vi "PID Test.vi"() -> ()   [LabVIEW 2017]
uses:
  <vilib>/addons/control/pid/NI_PID_pid.lvlib
  <vilib>/addons/control/pid/pid.llb/PID (DBL).vi
  <vilib>/myRIO/Instrument Drivers/Utilities/Utilities.lvlib
panel:
  out "Time (s)":dbl
  out "Output String":string
  out "PID Output":dbl(graph)
  out "SP & PV":T1(graph)
  out "Speed (mm/s)":dbl
  in  "PID gains":T2={"proportional gain (Kc)"=1.0, "integral time (Ti, min)"=0.01, "derivative time (Td, min)"=0.0} {"derivative time (Td, min)" format="%.3f"; "integral time (Ti, min)" format="%.3f"; "proportional gain (Kc)" format="%.3f"}
  out "dt out (s)":dbl format="%.3f"
  in  "FWD/RVS":bool
  in  "Frequency":dbl
  in  "Velocity Set Pt":dbl
  in  "stop":bool
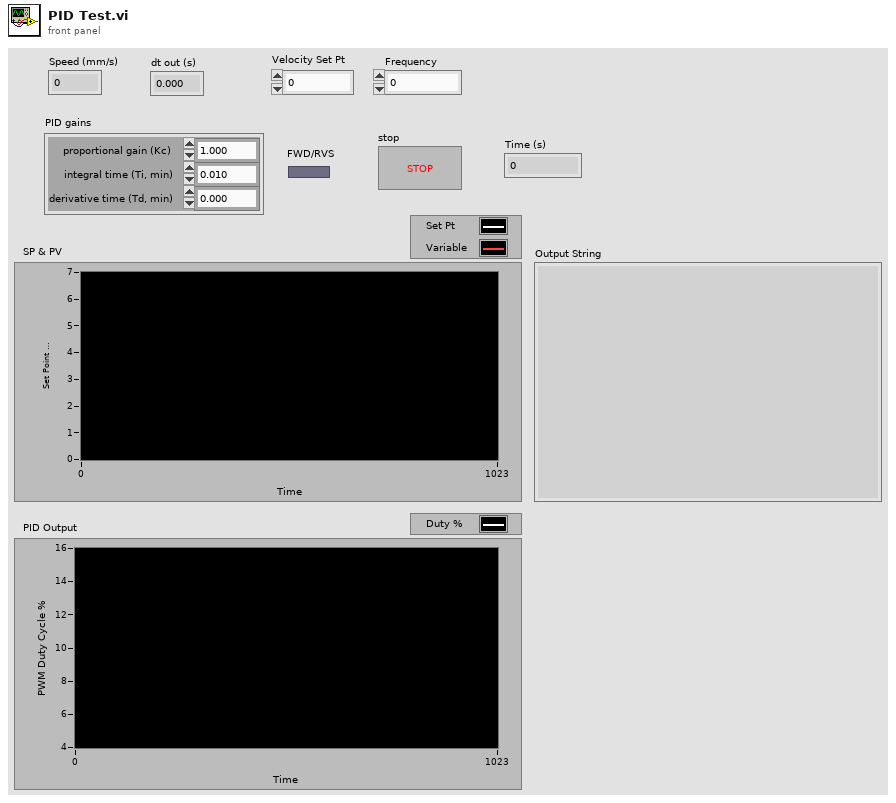
[diagram p1: front panel]
types:
  T1 = cluster{"Velocity Set Pt":dbl, "Velocity (mm/s)":dbl}
  T2 = cluster{"proportional gain (Kc)":dbl, "integral time (Ti, min)":dbl, "derivative time (Td, min)":dbl}
  T3 = typedef "Encoder Cluster.ctl" = cluster{"Y-axis rev count":dbl, "Y-axis distance":dbl, "X-axis rev count":dbl, "X-axis distance":dbl, "Y-axis direction":T4, "X-axis direction":T4, "X-counter val":i32, "Y-counter val":i32}
  T4 = typedef "Encoder Count Direction Enum.ctl" = enum16{"Counting Up", "Counting Down"}
  T5 = cluster{dbl, "Velocity Set Pt":dbl, dbl, "output":dbl, "proportional gain (Kc)":dbl, "integral time (Ti, min)":dbl, "derivative time (Td, min)":dbl}
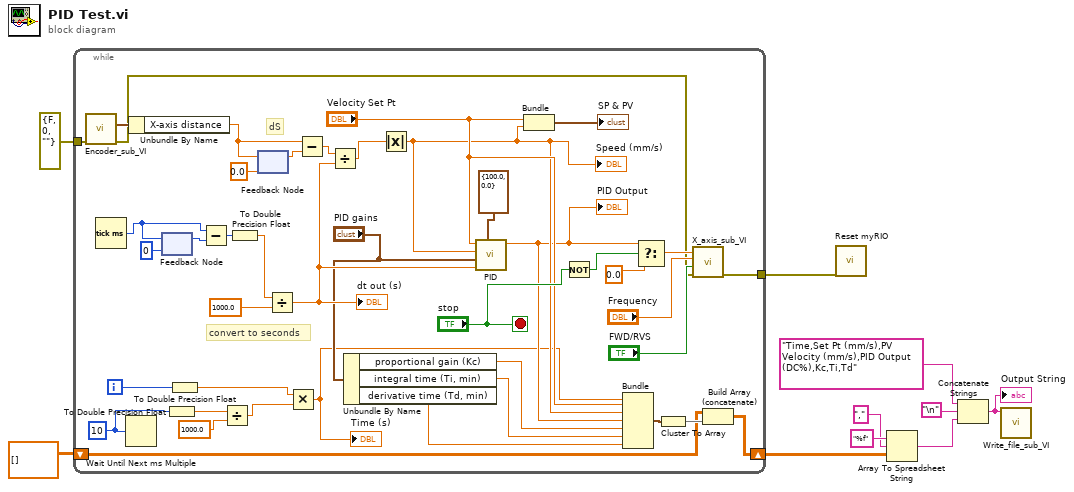
[diagram p0: block diagram]
diagram:
  n1 = while {
    shift-right: [w24] -> w3
    shift-left: dbl[][] [] ("element") -> [w25]
    tunnel: errorcluster {"status"=FALSE, "code"=0, "source"=""} ("error constant") -> [w23]
    tunnel: [w21] -> w1
    i -> [w13]
    stop <- "stop" stop-if-true
    w11 = u32 10 ("millisecond multiple")
    # "dS"
    # "convert to seconds"
    n2 = call "Encoder_sub_VI.vi"("error in (no error)"=w23) -> ("error out"=w22:errorcluster, "Encoder Output"=w50:T3)  [unwired: 9 in]
    n3 = Tick Count (ms)() -> (millisecond timer value=w35:u32)
    n4 = Wait Until Next ms Multiple(millisecond multiple=w11) -> ()  [unwired: 1 out]
    n5 = Unbundle By Name(w50) -> ("X-axis distance"=w46:dbl)
    n6 = feedback #1(u32 0 ("X-axis distance")) -> (w37:u32)
    n7 = feedback-in #1(w35) -> ()
    n8 = To Double Precision Float(number=w11) -> (double precision float=w20:dbl)
    n9 = To Double Precision Float(number=w13) -> (double precision float=w12:dbl)
    n10 = Subtract(x=w35, y=w37) -> (x-y=w34:u32)
    n11 = Divide(x=w20, y=1000.0) -> (x/y=w15:dbl)
    n12 = To Double Precision Float(number=w34) -> (double precision float=w33:dbl)
    n13 = feedback-in #2(w46) -> ()
    n14 = feedback #2(0.0 ("X-axis distance")) -> (w48:dbl)
    n15 = Divide(x=w33, y=1000.0) -> (x/y=w32:dbl)
    "dt out (s)" <- w32
    n16 = Multiply(x=w12, y=w15) -> (x*y=w14:dbl)
    "Time (s)" <- w14
    n17 = Subtract(x=w46, y=w48) -> (x-y=w45:dbl)
    n18 = Divide(x=w45, y=w32) -> (x/y=w44:dbl)
    n19 = Unbundle By Name("PID gains") -> ("proportional gain (Kc)"=w18:dbl, "integral time (Ti, min)"=w17:dbl, "derivative time (Td, min)"=w16:dbl)
    n20 = Absolute Value(x=w44) -> (abs(x)=w30:dbl)
    "Speed (mm/s)" <- w30
    n21 = call-poly <vilib>:"PID.vi"("output range"=cluster{"output high":dbl, "output low":dbl} {"output high"=100.0, "output low"=0.0}, "dt (s)"=w32, "PID gains"="PID gains", "process variable"=w30, "setpoint"="Velocity Set Pt") -> ("output"=w29:dbl)  [unwired: 5 in, 1 out]
    "PID Output" <- w29
    n22 = Bundle("Velocity Set Pt"="Velocity Set Pt", w30) -> (→"SP & PV":cluster{"Velocity Set Pt":dbl, dbl})  [unwired: 1 in]
    n23 = Not(x="stop") -> (.not. x?=w42:bool)
    n24 = Bundle(w14, "Velocity Set Pt"="Velocity Set Pt", w30, "output"=w29, "proportional gain (Kc)"=w18, "integral time (Ti, min)"=w17, "derivative time (Td, min)"=w16) -> (w27:T5)  [unwired: 1 in]
    n25 = Select(t=w29, s=w42, f=0.0) -> (s? t:f=w40:dbl)
    n26 = Cluster To Array(cluster=w27) -> (array=w26:dbl[])
    n27 = call "X_axis_sub_VI.vi"("error in (no error)"=w22, "FWD/RVS"="FWD/RVS", "Frequency"="Frequency", "Duty Cycle %"=w40) -> ("error out"=w21:errorcluster)  [unwired: 7 in]
    n28 = Build Array (concatenate)(w25, w26) -> (w24:dbl[][])
  }
  n29 = call <vilib>:"Reset myRIO.vi"("error in (no error)"=w1) -> ()  [unwired: 10 in, 1 out]
  n30 = Array To Spreadsheet String(delimiter (Tab)=",", array=w3, 3:"%f" ("format string")) -> (spreadsheet string=w9:string)
  n31 = Concatenate Strings("Time,Set Pt (mm/s),PV Velocity (mm/s),PID Output (DC%),Kc,Ti,Td", "\n", w9) -> (w8:string)
  "Output String" <- w8
  n32 = call "Write_file_sub_VI.vi"("Output String"=w8) -> ()  [unwired: 9 in, 2 out]
